vi "Aufschaltung CalGas Span.vi"(4 "Status Str Referenz":refnum<vi>, 6 "Sprachliste":string[][](array[string]), 7 "GD SPAN Eingänge":i32, 8 "error in (no error)":errorcluster caption="Fehler (Eingang, kein Fehler)", 9 "Component Index":i32, 10 "SPAN Index":i32, 11 "SpanInletClusterArray":T1[](array[typedef]) {"zusätzliche Zeitdauer Erster Punkt" min=30 step=1 format="%#_5g"; "Zeitdauer Stufen" format="%#_5g"; "Max Fehler" format="%#_5g"; "Anzahl Stufen" format="%#_5g"; "Komponenten"."Komponente 5"."Komponente:" items=["NO (350,3000) LP 191C", "NO2 (150) LP 191C (1of2)", "NO2 (2000) LP 191C (2of2)", "N2O (300) LP 191C (1of2)", "NH3 (300) LP 191C (1of2)", "NH3 (900,3000) LP 191C (2of2)", "HNCO (400) 191C", "H2O% (30) LP 191C", "Formaldehyde (70,500) LP 191C", "CO2 low% (4) LP 191C (2of2)", "CO2% (20) LP 191C (1of2)", "CO (700) LP 191C (1of3)", "CO% (1) LP 191C (2of3)", "Propylene (1000) LP 191C", "Aromatic HC C7 (500) LP 191C", "Ethylene (1000) LP 191C", "CH4 (250) LP 191C (1of2)", "CH4 (5000) LP 191C (2of2)", "Ethane (1000) LP 191C", "Acetylene (1000) LP 191C", "HNO2 (20) 191C", "MeOH (1000) 191C", "CO% (10) LP 191C (3of3)", "Formic Acid (100) 191C", "SO2 (500) LP 191C", "Acetaldehyde (1000) LP 191C", "COS (100) LP 191C", "1,3 butadiene (100) LP 191C", "Oil as Octane (200) LP 191C", "N2O (1000) LP 191C (2of2)", "Propane (200) LP 191C", "NO2 autorange (2000)", "CO autorange (100000)", "CH4 autorange (5000)", "NH3 autorange (3000)", "Temp. Gascell", "Pressure Gascell", "sBeam@2500"]; "Komponenten"."Komponente 5"."Konzentration IST" format="%#.4f"; "Komponenten"."Komponente 5"."Genauigkeit" format="%#.1f"; "Komponenten"."Komponente 4"."Komponente:" items=["NO (350,3000) LP 191C", "NO2 (150) LP 191C (1of2)", "NO2 (2000) LP 191C (2of2)", "N2O (300) LP 191C (1of2)", "NH3 (300) LP 191C (1of2)", "NH3 (900,3000) LP 191C (2of2)", "HNCO (400) 191C", "H2O% (30) LP 191C", "Formaldehyde (70,500) LP 191C", "CO2 low% (4) LP 191C (2of2)", "CO2% (20) LP 191C (1of2)", "CO (700) LP 191C (1of3)", "CO% (1) LP 191C (2of3)", "Propylene (1000) LP 191C", "Aromatic HC C7 (500) LP 191C", "Ethylene (1000) LP 191C", "CH4 (250) LP 191C (1of2)", "CH4 (5000) LP 191C (2of2)", "Ethane (1000) LP 191C", "Acetylene (1000) LP 191C", "HNO2 (20) 191C", "MeOH (1000) 191C", "CO% (10) LP 191C (3of3)", "Formic Acid (100) 191C", "SO2 (500) LP 191C", "Acetaldehyde (1000) LP 191C", "COS (100) LP 191C", "1,3 butadiene (100) LP 191C", "Oil as Octane (200) LP 191C", "N2O (1000) LP 191C (2of2)", "Propane (200) LP 191C", "NO2 autorange (2000)", "CO autorange (100000)", "CH4 autorange (5000)", "NH3 autorange (3000)", "Temp. Gascell", "Pressure Gascell", "sBeam@2500"]; "Komponenten"."Komponente 4"."Konzentration IST" format="%#.4f"; "Komponenten"."Komponente 4"."Genauigkeit" format="%#.1f"; "Komponenten"."Komponente 3"."Komponente:" items=["NO (350,3000) LP 191C", "NO2 (150) LP 191C (1of2)", "NO2 (2000) LP 191C (2of2)", "N2O (300) LP 191C (1of2)", "NH3 (300) LP 191C (1of2)", "NH3 (900,3000) LP 191C (2of2)", "HNCO (400) 191C", "H2O% (30) LP 191C", "Formaldehyde (70,500) LP 191C", "CO2 low% (4) LP 191C (2of2)", "CO2% (20) LP 191C (1of2)", "CO (700) LP 191C (1of3)", "CO% (1) LP 191C (2of3)", "Propylene (1000) LP 191C", "Aromatic HC C7 (500) LP 191C", "Ethylene (1000) LP 191C", "CH4 (250) LP 191C (1of2)", "CH4 (5000) LP 191C (2of2)", "Ethane (1000) LP 191C", "Acetylene (1000) LP 191C", "HNO2 (20) 191C", "MeOH (1000) 191C", "CO% (10) LP 191C (3of3)", "Formic Acid (100) 191C", "SO2 (500) LP 191C", "Acetaldehyde (1000) LP 191C", "COS (100) LP 191C", "1,3 butadiene (100) LP 191C", "Oil as Octane (200) LP 191C", "N2O (1000) LP 191C (2of2)", "Propane (200) LP 191C", "NO2 autorange (2000)", "CO autorange (100000)", "CH4 autorange (5000)", "NH3 autorange (3000)", "Temp. Gascell", "Pressure Gascell", "sBeam@2500"]; "Komponenten"."Komponente 3"."Konzentration IST" format="%#.4f"; "Komponenten"."Komponente 3"."Genauigkeit" format="%#.1f"; "Komponenten"."Komponente 2"."Komponente:" items=["NO (350,3000) LP 191C", "NO2 (150) LP 191C (1of2)", "NO2 (2000) LP 191C (2of2)", "N2O (300) LP 191C (1of2)", "NH3 (300) LP 191C (1of2)", "NH3 (900,3000) LP 191C (2of2)", "HNCO (400) 191C", "H2O% (30) LP 191C", "Formaldehyde (70,500) LP 191C", "CO2 low% (4) LP 191C (2of2)", "CO2% (20) LP 191C (1of2)", "CO (700) LP 191C (1of3)", "CO% (1) LP 191C (2of3)", "Propylene (1000) LP 191C", "Aromatic HC C7 (500) LP 191C", "Ethylene (1000) LP 191C", "CH4 (250) LP 191C (1of2)", "CH4 (5000) LP 191C (2of2)", "Ethane (1000) LP 191C", "Acetylene (1000) LP 191C", "HNO2 (20) 191C", "MeOH (1000) 191C", "CO% (10) LP 191C (3of3)", "Formic Acid (100) 191C", "SO2 (500) LP 191C", "Acetaldehyde (1000) LP 191C", "COS (100) LP 191C", "1,3 butadiene (100) LP 191C", "Oil as Octane (200) LP 191C", "N2O (1000) LP 191C (2of2)", "Propane (200) LP 191C", "NO2 autorange (2000)", "CO autorange (100000)", "CH4 autorange (5000)", "NH3 autorange (3000)", "Temp. Gascell", "Pressure Gascell", "sBeam@2500"]; "Komponenten"."Komponente 2"."Konzentration IST" format="%#.4f"; "Komponenten"."Komponente 2"."Genauigkeit" format="%#.1f"; "Komponenten"."Komponente 1"."Komponente:" items=["NO (350,3000) LP 191C", "NO2 (150) LP 191C (1of2)", "NO2 (2000) LP 191C (2of2)", "N2O (300) LP 191C (1of2)", "NH3 (300) LP 191C (1of2)", "NH3 (900,3000) LP 191C (2of2)", "HNCO (400) 191C", "H2O% (30) LP 191C", "Formaldehyde (70,500) LP 191C", "CO2 low% (4) LP 191C (2of2)", "CO2% (20) LP 191C (1of2)", "CO (700) LP 191C (1of3)", "CO% (1) LP 191C (2of3)", "Propylene (1000) LP 191C", "Aromatic HC C7 (500) LP 191C", "Ethylene (1000) LP 191C", "CH4 (250) LP 191C (1of2)", "CH4 (5000) LP 191C (2of2)", "Ethane (1000) LP 191C", "Acetylene (1000) LP 191C", "HNO2 (20) 191C", "MeOH (1000) 191C", "CO% (10) LP 191C (3of3)", "Formic Acid (100) 191C", "SO2 (500) LP 191C", "Acetaldehyde (1000) LP 191C", "COS (100) LP 191C", "1,3 butadiene (100) LP 191C", "Oil as Octane (200) LP 191C", "N2O (1000) LP 191C (2of2)", "Propane (200) LP 191C", "NO2 autorange (2000)", "CO autorange (100000)", "CH4 autorange (5000)", "NH3 autorange (3000)", "Temp. Gascell", "Pressure Gascell", "sBeam@2500"]; "Komponenten"."Komponente 1"."Konzentration IST" format="%#.4f"; "Komponenten"."Komponente 1"."Genauigkeit" format="%#.1f"; "Ablaufdatum" format="%<%d.%m.%Y>T"; "Gasflasche" items=["----"=10000, "IAG NH3 3000"=0, "IAG NH3 200"=1, "IAG NH3 2000"=2, "IAG MG"=3, "IAG O2"=4]}) -> (0 "error out":errorcluster caption="Fehler (Ausgang)", 1 "Status out":string, 2 "SPAN Index out":i32, 3 "SpanInletClusterArray out":T1[](array[typedef]) {"zusätzliche Zeitdauer Erster Punkt" min=30 step=1 format="%#_5g"; "Zeitdauer Stufen" format="%#_5g"; "Max Fehler" format="%#_5g"; "Anzahl Stufen" format="%#_5g"; "Komponenten"."Komponente 5"."Komponente:" items=["NO (350,3000) LP 191C", "NO2 (150) LP 191C (1of2)", "NO2 (2000) LP 191C (2of2)", "N2O (300) LP 191C (1of2)", "NH3 (300) LP 191C (1of2)", "NH3 (900,3000) LP 191C (2of2)", "HNCO (400) 191C", "H2O% (30) LP 191C", "Formaldehyde (70,500) LP 191C", "CO2 low% (4) LP 191C (2of2)", "CO2% (20) LP 191C (1of2)", "CO (700) LP 191C (1of3)", "CO% (1) LP 191C (2of3)", "Propylene (1000) LP 191C", "Aromatic HC C7 (500) LP 191C", "Ethylene (1000) LP 191C", "CH4 (250) LP 191C (1of2)", "CH4 (5000) LP 191C (2of2)", "Ethane (1000) LP 191C", "Acetylene (1000) LP 191C", "HNO2 (20) 191C", "MeOH (1000) 191C", "CO% (10) LP 191C (3of3)", "Formic Acid (100) 191C", "SO2 (500) LP 191C", "Acetaldehyde (1000) LP 191C", "COS (100) LP 191C", "1,3 butadiene (100) LP 191C", "Oil as Octane (200) LP 191C", "N2O (1000) LP 191C (2of2)", "Propane (200) LP 191C", "NO2 autorange (2000)", "CO autorange (100000)", "CH4 autorange (5000)", "NH3 autorange (3000)", "Temp. Gascell", "Pressure Gascell", "sBeam@2500"]; "Komponenten"."Komponente 5"."Konzentration IST" format="%#.4f"; "Komponenten"."Komponente 5"."Genauigkeit" format="%#.1f"; "Komponenten"."Komponente 4"."Komponente:" items=["NO (350,3000) LP 191C", "NO2 (150) LP 191C (1of2)", "NO2 (2000) LP 191C (2of2)", "N2O (300) LP 191C (1of2)", "NH3 (300) LP 191C (1of2)", "NH3 (900,3000) LP 191C (2of2)", "HNCO (400) 191C", "H2O% (30) LP 191C", "Formaldehyde (70,500) LP 191C", "CO2 low% (4) LP 191C (2of2)", "CO2% (20) LP 191C (1of2)", "CO (700) LP 191C (1of3)", "CO% (1) LP 191C (2of3)", "Propylene (1000) LP 191C", "Aromatic HC C7 (500) LP 191C", "Ethylene (1000) LP 191C", "CH4 (250) LP 191C (1of2)", "CH4 (5000) LP 191C (2of2)", "Ethane (1000) LP 191C", "Acetylene (1000) LP 191C", "HNO2 (20) 191C", "MeOH (1000) 191C", "CO% (10) LP 191C (3of3)", "Formic Acid (100) 191C", "SO2 (500) LP 191C", "Acetaldehyde (1000) LP 191C", "COS (100) LP 191C", "1,3 butadiene (100) LP 191C", "Oil as Octane (200) LP 191C", "N2O (1000) LP 191C (2of2)", "Propane (200) LP 191C", "NO2 autorange (2000)", "CO autorange (100000)", "CH4 autorange (5000)", "NH3 autorange (3000)", "Temp. Gascell", "Pressure Gascell", "sBeam@2500"]; "Komponenten"."Komponente 4"."Konzentration IST" format="%#.4f"; "Komponenten"."Komponente 4"."Genauigkeit" format="%#.1f"; "Komponenten"."Komponente 3"."Komponente:" items=["NO (350,3000) LP 191C", "NO2 (150) LP 191C (1of2)", "NO2 (2000) LP 191C (2of2)", "N2O (300) LP 191C (1of2)", "NH3 (300) LP 191C (1of2)", "NH3 (900,3000) LP 191C (2of2)", "HNCO (400) 191C", "H2O% (30) LP 191C", "Formaldehyde (70,500) LP 191C", "CO2 low% (4) LP 191C (2of2)", "CO2% (20) LP 191C (1of2)", "CO (700) LP 191C (1of3)", "CO% (1) LP 191C (2of3)", "Propylene (1000) LP 191C", "Aromatic HC C7 (500) LP 191C", "Ethylene (1000) LP 191C", "CH4 (250) LP 191C (1of2)", "CH4 (5000) LP 191C (2of2)", "Ethane (1000) LP 191C", "Acetylene (1000) LP 191C", "HNO2 (20) 191C", "MeOH (1000) 191C", "CO% (10) LP 191C (3of3)", "Formic Acid (100) 191C", "SO2 (500) LP 191C", "Acetaldehyde (1000) LP 191C", "COS (100) LP 191C", "1,3 butadiene (100) LP 191C", "Oil as Octane (200) LP 191C", "N2O (1000) LP 191C (2of2)", "Propane (200) LP 191C", "NO2 autorange (2000)", "CO autorange (100000)", "CH4 autorange (5000)", "NH3 autorange (3000)", "Temp. Gascell", "Pressure Gascell", "sBeam@2500"]; "Komponenten"."Komponente 3"."Konzentration IST" format="%#.4f"; "Komponenten"."Komponente 3"."Genauigkeit" format="%#.1f"; "Komponenten"."Komponente 2"."Komponente:" items=["NO (350,3000) LP 191C", "NO2 (150) LP 191C (1of2)", "NO2 (2000) LP 191C (2of2)", "N2O (300) LP 191C (1of2)", "NH3 (300) LP 191C (1of2)", "NH3 (900,3000) LP 191C (2of2)", "HNCO (400) 191C", "H2O% (30) LP 191C", "Formaldehyde (70,500) LP 191C", "CO2 low% (4) LP 191C (2of2)", "CO2% (20) LP 191C (1of2)", "CO (700) LP 191C (1of3)", "CO% (1) LP 191C (2of3)", "Propylene (1000) LP 191C", "Aromatic HC C7 (500) LP 191C", "Ethylene (1000) LP 191C", "CH4 (250) LP 191C (1of2)", "CH4 (5000) LP 191C (2of2)", "Ethane (1000) LP 191C", "Acetylene (1000) LP 191C", "HNO2 (20) 191C", "MeOH (1000) 191C", "CO% (10) LP 191C (3of3)", "Formic Acid (100) 191C", "SO2 (500) LP 191C", "Acetaldehyde (1000) LP 191C", "COS (100) LP 191C", "1,3 butadiene (100) LP 191C", "Oil as Octane (200) LP 191C", "N2O (1000) LP 191C (2of2)", "Propane (200) LP 191C", "NO2 autorange (2000)", "CO autorange (100000)", "CH4 autorange (5000)", "NH3 autorange (3000)", "Temp. Gascell", "Pressure Gascell", "sBeam@2500"]; "Komponenten"."Komponente 2"."Konzentration IST" format="%#.4f"; "Komponenten"."Komponente 2"."Genauigkeit" format="%#.1f"; "Komponenten"."Komponente 1"."Komponente:" items=["NO (350,3000) LP 191C", "NO2 (150) LP 191C (1of2)", "NO2 (2000) LP 191C (2of2)", "N2O (300) LP 191C (1of2)", "NH3 (300) LP 191C (1of2)", "NH3 (900,3000) LP 191C (2of2)", "HNCO (400) 191C", "H2O% (30) LP 191C", "Formaldehyde (70,500) LP 191C", "CO2 low% (4) LP 191C (2of2)", "CO2% (20) LP 191C (1of2)", "CO (700) LP 191C (1of3)", "CO% (1) LP 191C (2of3)", "Propylene (1000) LP 191C", "Aromatic HC C7 (500) LP 191C", "Ethylene (1000) LP 191C", "CH4 (250) LP 191C (1of2)", "CH4 (5000) LP 191C (2of2)", "Ethane (1000) LP 191C", "Acetylene (1000) LP 191C", "HNO2 (20) 191C", "MeOH (1000) 191C", "CO% (10) LP 191C (3of3)", "Formic Acid (100) 191C", "SO2 (500) LP 191C", "Acetaldehyde (1000) LP 191C", "COS (100) LP 191C", "1,3 butadiene (100) LP 191C", "Oil as Octane (200) LP 191C", "N2O (1000) LP 191C (2of2)", "Propane (200) LP 191C", "NO2 autorange (2000)", "CO autorange (100000)", "CH4 autorange (5000)", "NH3 autorange (3000)", "Temp. Gascell", "Pressure Gascell", "sBeam@2500"]; "Komponenten"."Komponente 1"."Konzentration IST" format="%#.4f"; "Komponenten"."Komponente 1"."Genauigkeit" format="%#.1f"; "Ablaufdatum" format="%<%d.%m.%Y>T"; "Gasflasche" items=["----"=10000, "IAG NH3 3000"=0, "IAG NH3 200"=1, "IAG NH3 2000"=2, "IAG MG"=3, "IAG O2"=4]})   [LabVIEW 2020, in "Linearisierung v2.lvlib" / "SpanEinstellungen.lvlib"]
uses:
  SpanEinstellungen.lvlib
  SpanInletCluster.ctl
  Seiten/System Einstellungen V2/Konfig Gasflasche.ctl
  Seiten/System Einstellungen V2/Analysatoren.ctl
  Seiten/System Einstellungen V2/Gasflasche Auswahl.ctl
  Komponentencluster mit Formel.ctl
  Komponentenauswahl mit Formel.ctl
  Visualisierungs Elemente/String - Eingabefeld.ctl
  Einheit.ctl
  Seiten/System Einstellungen V2/Traegergas.ctl
  Aktion Lin Daten aufarbeiten.ctl
  Visualisierungs Elemente/Zahlen-Eingabefeld.ctl
  Seiten/CalGas Aufschaltung/FGV CalGas Aktionen.ctl
  Seiten/CalGas Aufschaltung/Auswahl Aufschaltpunkt.ctl
  Gasteiler/Aktionen FGV Gasteiler Daten.ctl
  Aktion FGV GD Errors sammeln.ctl
  GD Info Cluster.ctl
  LIN ErrorCluster.ctl
  Gasteiler/AK-Komm Gasteiler/Aktionen AK Komm.ctl
  Gasteiler/HovaCAL_Interface/Kommunikation/Aktion_FGV_HovaCAL_Interface_GetData.ctl
  Gasteiler/HovaCAL_Interface/Kommunikation/Aktion FGV HovaCAL Interface Autolin.ctl
  Kalibrier Info Cluster.ctl
  Funktionstasten/Funktionstasten-Aktion.ctl
  Funktionstasten/Zustaende.ctl
  Seiten/EL3000/FID/FID Kalibrierung/FID Kalibrieren.ctl
  Seiten/EL3000/PMA/Kalibrieren/Kalibrierung O2.ctl
  Seiten/CalGas Aufschaltung/CalGas Aufschaltung.lvlib
  Seiten/System Einstellungen V2/System Einstellungen V2.lvlib
  Gasteiler/AK-Komm Gasteiler/Alter Gasteiler/Alter Gasteiler.lvlib
  Gasteiler/AK-Komm Gasteiler/Alter Gasteiler/Aktionen AK Komm_ALT.ctl
  Gasteiler/AK-Komm Gasteiler/AK Komm Gasteiler.lvlib
  Gasteiler/Horiba/Aktion Befehl.ctl
  Gasteiler/Horiba/Horiba GDC.lvlib
  Gasteiler/Gasteiler.lvlib
  Linearisierung v2.lvlib
  Funktionstasten/Funktionstasten.lvlib
  Seiten/EL3000/PMA/Kalibrieren/Kalibrieren.lvlib
  Seiten/EL3000/Allgemeine VI/Allgemeine VI.lvlib
  Seiten/EL3000/FID/FID Kalibrierung/FID Kalibrierung.lvlib
  Gasteiler/HovaCAL_Interface/Kommunikation/Kommunikation.lvlib
panel:
  # "sec"
  # "%"
  # "sec"
  # "Komponente"
  # "Formel"
  # "Konzentration"
  # "Einheit"
  # "Genauigkeit [%]"
  # "sec"
  # "%"
  # "sec"
  # "Komponente"
  # "Formel"
  # "Konzentration"
  # "Einheit"
  # "Genauigkeit [%]"
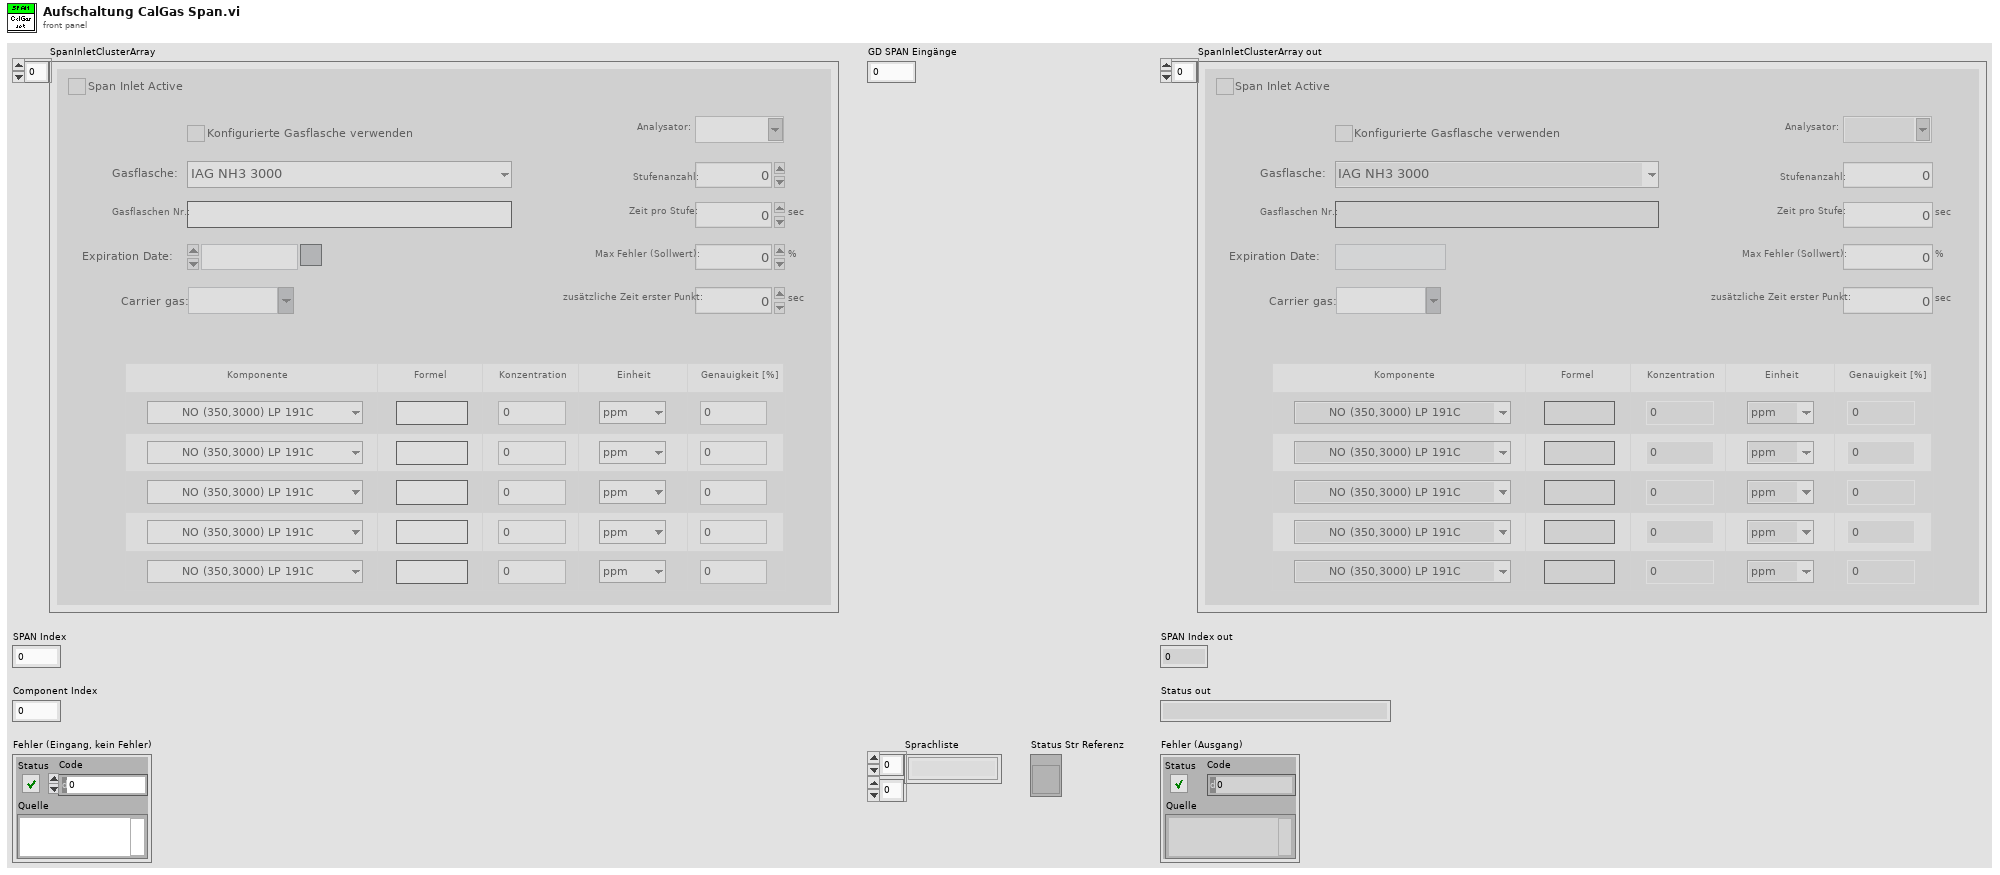
[diagram p1: front panel]
types:
  T1 = typedef "Linearisierung v2.lvlib/SpanEinstellungen.lvlib/SpanInletCluster.ctl" = cluster{"Span Inlet Active":T2, "Analysator":T3, "Konfig Gasflasche":T2, "Gasflasche":T4, "Gasflaschen Nr.:":string, "Ablaufdatum":timestamp, "Komponenten":T5, "Zeitdauer Stufen":sgl, "Max Fehler":sgl, "Anzahl Stufen":sgl, "Trägergas":T9, "zusätzliche Zeitdauer Erster Punkt":sgl}
  T2 = typedef "System Einstellungen V2.lvlib/Konfig Gasflasche.ctl" = bool
  T3 = typedef "System Einstellungen V2.lvlib/Analysatoren.ctl" = string
  T4 = typedef "System Einstellungen V2.lvlib/Gasflasche Auswahl.ctl" = u16
  T5 = typedef "Linearisierung v2.lvlib/SpanEinstellungen.lvlib/Komponentencluster mit Formel.ctl" = cluster{"Komponente 1":T6, "Komponente 2":T6, "Komponente 3":T6, "Komponente 4":T6, "Komponente 5":T6}
  T6 = typedef "Linearisierung v2.lvlib/SpanEinstellungen.lvlib/Komponentenauswahl mit Formel.ctl" = cluster{"Komponente:":u16, "Summenformel":T7, "Konzentration IST":dbl, "Einheit":T8, "Genauigkeit":dbl}
  T7 = typedef "String - Eingabefeld.ctl" = string
  T8 = typedef "Linearisierung v2.lvlib/SpanEinstellungen.lvlib/Einheit.ctl" = enum16{"ppm", "%"}
  T9 = typedef "System Einstellungen V2.lvlib/Traegergas.ctl" = string
  T10 = typedef "Zahlen-Eingabefeld.ctl" = sgl
  T11 = typedef "Linearisierung v2.lvlib/Aktion Lin Daten aufarbeiten.ctl" = enum16{"lesen", "Protkolldaten", "speichern", "laden", "EPA auswerten", "Tabelle schreiben", "Lin auswerten", "Tab init", "Stufentabelle", "EPA aktiviert", "Nachbehandlung laden", "Tabelle löschen", "Istwerte löschen", "Zeile löschen", "Zeile einfügen", "LIN aktiviert", "LIN/EPA aktiv laden", "EGAK Tab", "LIN übernehmen", "Tab init ohne Stufen"}
  T12 = typedef "Linearisierung v2.lvlib/Lin-Polynom Daten.ctl" = cluster{"Messgerät":string, "Kalibrator (Gasteiler)":string, "Bearbeiter/in":string, "Komponente":string, "Zeitstempel":timestamp, "F_max gefordert (%)":sgl, "F_max in %":sgl, "F_max in ppm":sgl, "Vorschlag Ordnung":i32, "Polynom OK":bool, "Polynomkoeff.":dbl[], "Prüfgas Konzentration":dbl, "Pfad EPA":string, "Pfad_LIN":string, "Gasnummer:":u8, "Komponentenauswahl":T13, "Verdünnungsgas":T15, "Zeitdauer Stufe":T10, "Anzahl Stufen":T10, "F_max in % EPA":sgl, "F_max in ppm EPA":sgl, "F_max in % LIN":sgl, "F_max in ppm LIN":sgl, "Punkte umkehren":bool, "EPA Optionsfeld":T16, "Autolin Hovacal":T17, "Spanfactors":sgl[], "Kalibrierauswahl":T18, "Conditions:":T19, "Gasflaschen Nr.:":string, "Bottle Accuracy":dbl, "Konfig Gasflasche":T2, "Gasflasche":T4, "HovaCAL Flow AutoLin":T20, "MFC Output":T21, "Gas Ablaufdatum":timestamp, "Lin Modus":T22, "zusätzliche Zeitdauer Erster Punkt":sgl, "Offsets":sgl[]}
  T13 = typedef "Linearisierung v2.lvlib/KomponentenArray.ctl" = cluster{"Komponente:":T14, "Konzentration":dbl}[]
  T14 = typedef "Auswahlfeld.ctl" = u16
  T15 = typedef "Linearisierung v2.lvlib/Gasteiler.lvlib/Prüfgas in.ctl" = u16
  T16 = typedef "Linearisierung v2.lvlib/EPA Optionsfeld.ctl" = enum32{"Istwert", "Rohwert", "Linearisierter Wert"}
  T17 = typedef "Linearisierung v2.lvlib/Gasteiler.lvlib/HovaCal.lvlib/AutoLin Hovacal.ctl" = enum32{"Keine Auswahl", "Optionsauswahl 1", "Optionsauswahl 2"}
  T18 = typedef "Linearisierung v2.lvlib/Kalibrieroption.ctl" = u16
  T19 = typedef "Linearisierung v2.lvlib/Linearity verification 1065-307.lvlib/Condition.ctl" = u16
  T20 = typedef "Linearisierung v2.lvlib/Gasteiler.lvlib/HovaCAL_Interface.lvlib/Controls.lvlib/Flow Einstellung.ctl" = cluster{"HovaCAL Flow Input Cluster":dbl}
  T21 = typedef "Linearisierung v2.lvlib/Gasteiler.lvlib/HovaCAL_Interface.lvlib/Controls.lvlib/Pump state.ctl" = cluster{"Run":bool}
  T22 = typedef "CalGas Aufschaltung.lvlib/Lin Modus.ctl" = u16
  T23 = typedef "CalGas Aufschaltung.lvlib/FGV CalGas Aktionen.ctl" = enum16{"lesen", "Analysator Auswahl", "Def.CalGas", "Aufschaltung CalGas", "laden", "speichern", "KAL extrahieren"}
  T24 = typedef "CalGas Aufschaltung.lvlib/Auswahl Aufschaltpunkt.ctl" = enum16{"über Filterblock", "Analysator direkt", "über PNS", "Entnahme", "Gasdivider"}
  T25 = typedef "Linearisierung v2.lvlib/SpanEinstellungen.lvlib/GD Info Cluster.ctl" = cluster{"Wobei":string, "Status":string, "Errors":T26, "Empfangsdaten":string[], "Zeitstempel":string}
  T26 = typedef "Linearisierung v2.lvlib/LIN ErrorCluster.ctl" = cluster{"Störung Kommunikation":bool, "Pressure carrier gas":bool, "Pressure diluted gas":bool, "Outlet Pressure":bool, "SNOX before SAIR":bool, "Störung Gasteiler":bool}
  T27 = typedef "Linearisierung v2.lvlib/SpanEinstellungen.lvlib/Aktion FGV GD Errors sammeln.ctl" = enum16{"lesen", "init", "GD Infos sammeln", "Kalibrierinfos sammeln", "Test Data", "GD Infos selektiv sammeln"}
  T28 = typedef "Linearisierung v2.lvlib/Gasteiler.lvlib/Aktionen FGV Gasteiler Daten.ctl" = enum16{"lesen", "Gasteiler Daten", "Seriellen Param.", "MB-Endwert", "laden", "speichern", "Anforderung", "TCP", "Aufzeichnung Start"}
  T29 = typedef "Linearisierung v2.lvlib/Gasteiler.lvlib/AK Komm Gasteiler.lvlib/Aktionen AK Komm.ctl" = enum16{"lesen", "initialisieren", "beenden", "Status", "SMAN", "SREM", "STBY", "ASTF", "ASTZ", "SLST", "AGAT", "EGAK", "AGAK", "AKAK", "ADRU", "SKOP", "SVSA", "SVSZ", "SONO", "SAIR", "SNOX", "ANOX", "SSPL", "SRUC", "SLIN", "ALST", "ETYP", "SVIO", "LCYL", "CCYL", "DCYL", "SCYL", "GCYL", "DRGV", "DRDC"}
  T30 = typedef "Linearisierung v2.lvlib/Gasteiler.lvlib/AK Komm Gasteiler.lvlib/Alter Gasteiler.lvlib/Aktionen AK Komm_ALT.ctl" = enum16{"lesen", "initialisieren", "beenden", "SRES", "STBY", "SREM", "SMAN", "SLIN", "SLCH", "SLST", "SSPL", "AGAT", "ALST", "ASTZ", "ASTF", "AGAK", "EGAK"}
  T31 = typedef "Linearisierung v2.lvlib/Gasteiler.lvlib/Horiba GDC.lvlib/Aktion Befehl.ctl" = enum16{"lesen", "initialisieren", "Beenden", "Standby", "GD/CC", "Info", "Flow", "Alarm", "GD parameter", "GD point", "Durchfluss", "Spuelen1", "Spuelen1 On", "Spuelen1Off", "Spuelen2", "Ventil-Abfrage", "Reset"}
  T32 = typedef "Linearisierung v2.lvlib/Gasteiler.lvlib/HovaCAL_Interface.lvlib/Kommunikation.lvlib/Aktion_FGV_HovaCAL_Interface_GetData.ctl" = enum16{"lesen", "SystemInfo", "MFC Info", "actual Values", "Limits", "first contact"}
  T33 = typedef "Linearisierung v2.lvlib/Gasteiler.lvlib/HovaCAL_Interface.lvlib/Kommunikation.lvlib/Aktion FGV HovaCAL Interface Autolin.ctl" = enum16{"lesen", "schreiben", "MFC Komponente fix setzen", "init"}
  T34 = typedef "CalGas Aufschaltung.lvlib/Aufschaltung CalGas.ctl" = cluster{"Kalibriergas":T14, "Aufschaltpunkt":T24, "Analysator":T35}
  T35 = typedef "CalGas Aufschaltung.lvlib/Auswahl Analysator.ctl" = enum16{"FT-IR", "FID", "PMA", "PMA/FID/FT-IR"}
  T36 = typedef "Linearisierung v2.lvlib/GasteilerType.ctl" = u16
  T37 = typedef "Linearisierung v2.lvlib/Gasteiler.lvlib/Gasteiler Fehler.ctl" = cluster{"Pressure carrier gas":bool, "Pressure diluted gas":bool, "Outlet Pressure":bool, "SNOX before SAIR":bool}
  T38 = typedef "Linearisierung v2.lvlib/Gasteiler.lvlib/HovaCAL_Interface.lvlib/Controls.lvlib/Info Cluster.ctl" = cluster{"device":string, "version":string, "number of mfc":i32, "number of pumps":i32, "number of temp controllers":i32, "number of mfs":i32, "number of balances":i32}
  T39 = typedef "Funktionstasten.lvlib/Zustaende.ctl" = enum16{"Standby", "Pause", "Eco", "Messen", "Kalibrieren", "Spülen Filter", "Spülen Leitung", "Umgebungsluft", "0-Gas", "Cal-Gas", "CG zu PNS", "-------------", "Init 1", "Init 2", "Init 3", "Init 4", "Messen vorbereiten", "Messen durchführen", "Exit"}
  T40 = typedef "Funktionstasten.lvlib/Funktionstasten-Aktion.ctl" = enum16{"Initialisieren", "Zustand setzen", "Taste gedrückt", "Fehler speichern", "Lesen", "Manuell", "Remote", "Bitparallel", "Samplepoint", "Zeit Prüfen", "reset Umschalten"}
  T41 = typedef "ABB-EL3000.lvlib/FID.lvlib/FID Kalibrierung.lvlib/FID Kalibrieren.ctl" = enum16{"CH4 Nullpunkt", "THC Nullpunkt", "NMHC Nullpunkt", "CH4 Endpunkt", "THC Endpunkt", "NMHC Endpunkt"}
  T42 = typedef "ABB-EL3000.lvlib/PMA.lvlib/Kalibrieren.lvlib/Kalibrierung O2.ctl" = enum16{"Nullpunkt O2", "Endpunkt O2"}
  T43 = typedef "Linearisierung v2.lvlib/SpanEinstellungen.lvlib/Kalibrier Info Cluster.ctl" = cluster{"Wobei":string, "Calibration succesful":bool, "Value is in the valid range":bool, "Zeitstempel":string}
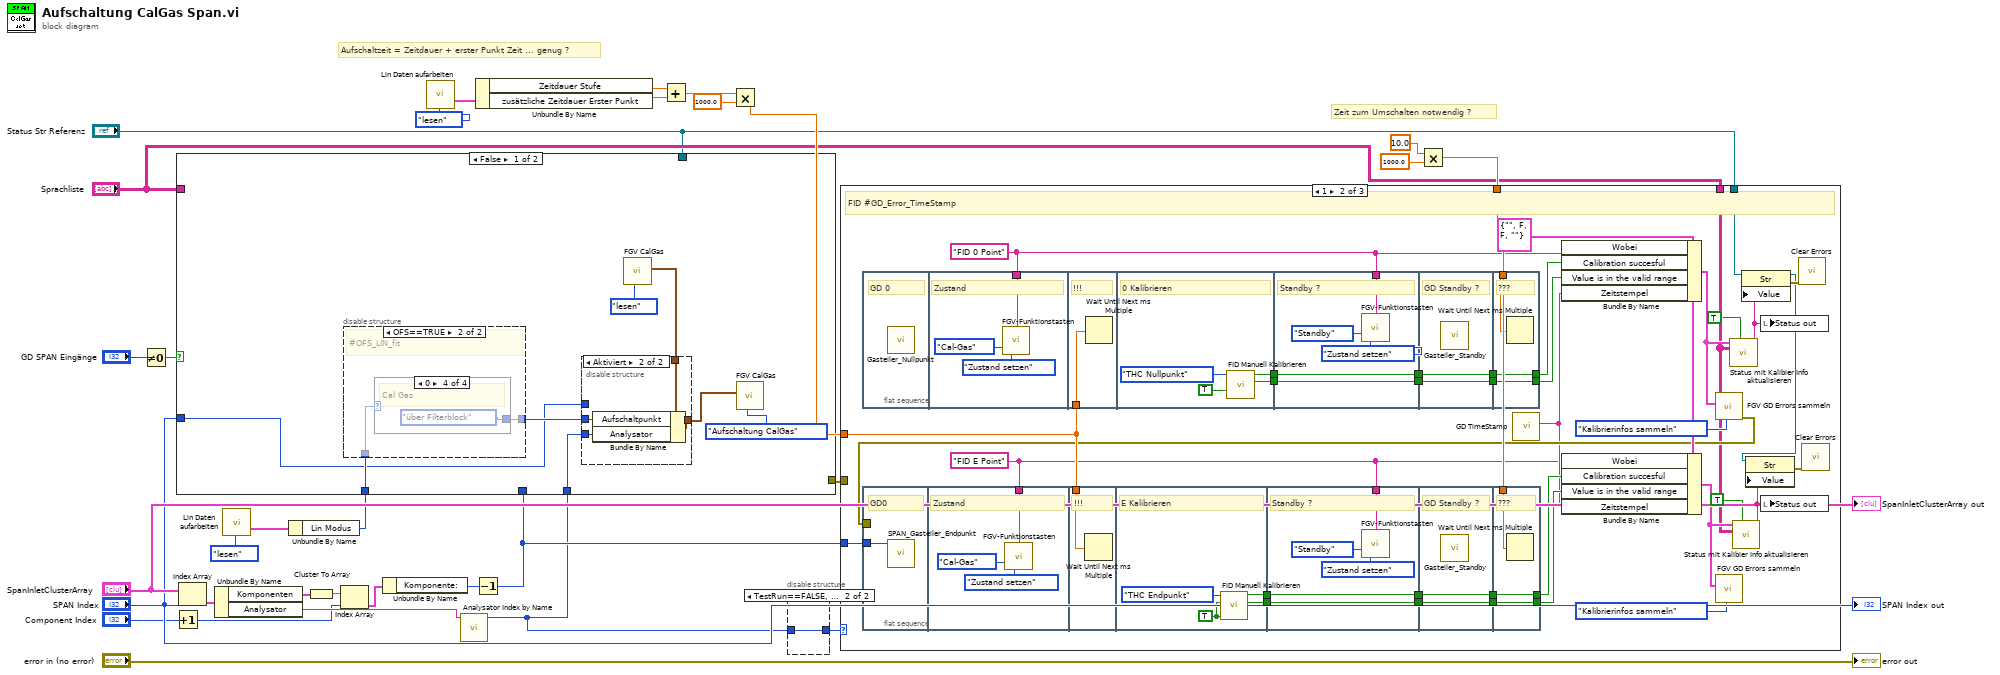
[diagram p0: block diagram]
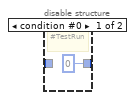
[diagram p2: hidden frame]
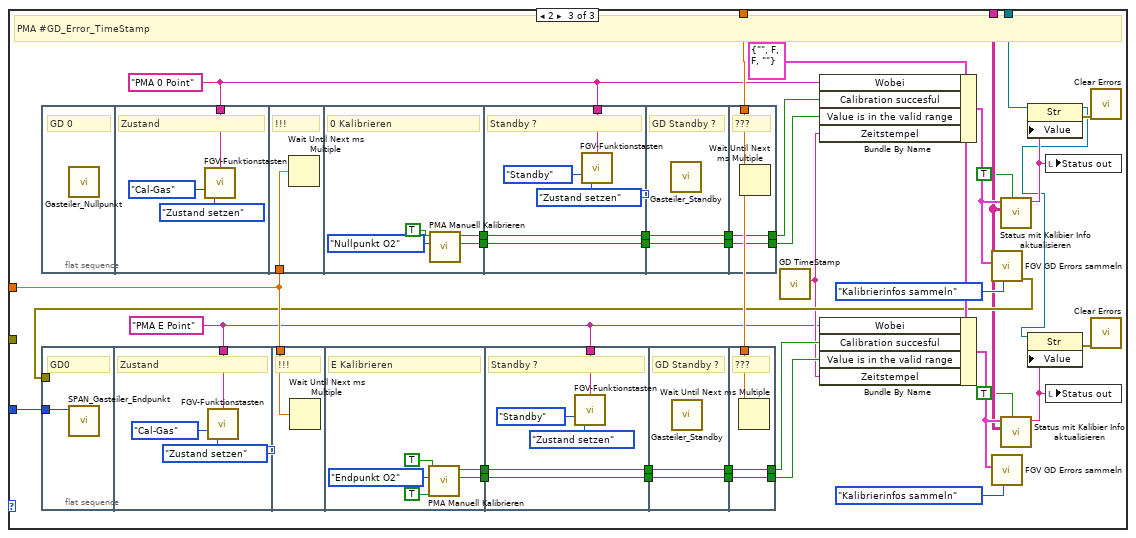
[diagram p4: hidden frame]
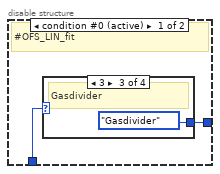
[diagram p5: hidden frame]
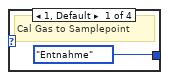
[diagram p6: hidden frame]
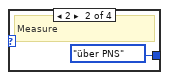
[diagram p7: hidden frame]
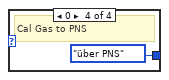
[diagram p8: hidden frame]
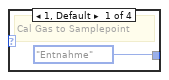
[diagram p9: hidden frame]
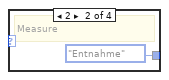
[diagram p10: hidden frame]
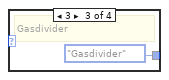
[diagram p11: hidden frame]
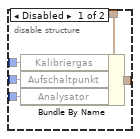
[diagram p12: hidden frame]
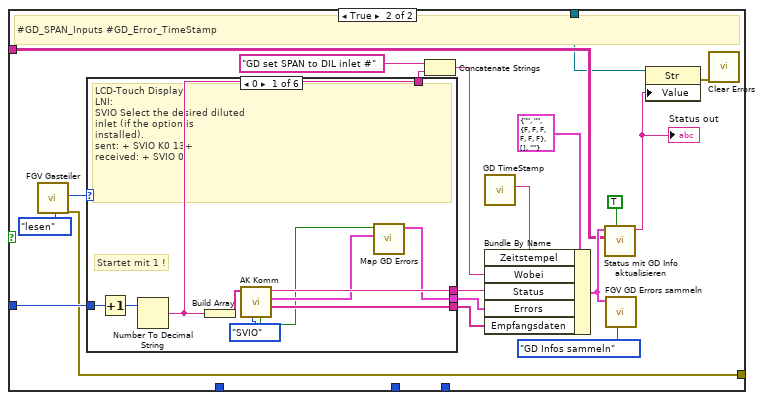
[diagram p13: hidden frame]
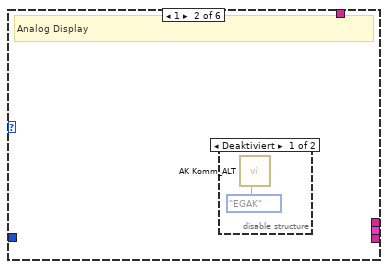
[diagram p14: hidden frame]
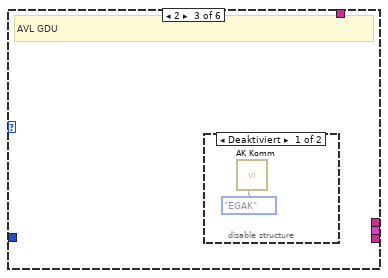
[diagram p16: hidden frame]
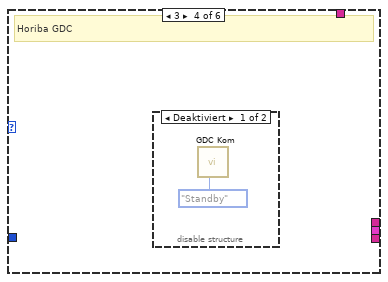
[diagram p18: hidden frame]
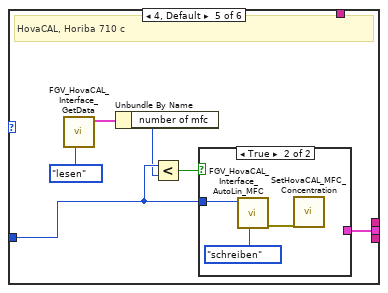
[diagram p20: hidden frame]
diagram:
  # "Zeit zum Umschalten notwendig ?"
  # "Aufschaltzeit = Zeitdauer + erster Punkt Zeit ... genug ?"
  n1 = Not Equal To 0?(x="GD SPAN Eingänge") -> (x != 0?=w28:bool)
  n2 = Increment(x="Component Index") -> (x+1=w17:i32)
  n3 = Index Array(array="SpanInletClusterArray", index="SPAN Index") -> (element=w23:T1)
  n4 = Unbundle By Name(w23) -> ("Komponenten"=w21:T5, "Analysator"=w31:T3)
  n5 = call "Lin Daten aufarbeiten.vi"("Aktionen"=Aktion_Lin_Daten_aufarbeiten."lesen") -> ("Lin-Polynom"=w26:T12)  [unwired: 16 in, 10 out]
  n6 = Unbundle By Name(w26) -> ("Lin Modus"=w2:T22)
  n7 = Cluster To Array(cluster=w21) -> (array=w22:T6[])
  n8 = Index Array(array=w22, index=w17) -> (element=w19:T6)
  n9 = Unbundle By Name(w19) -> ("Komponente:"=w18:u16)
  n10 = call "Lin Daten aufarbeiten.vi"("Aktionen"=Aktion_Lin_Daten_aufarbeiten."lesen") -> ("Lin-Polynom"=w14:T12)  [unwired: 16 in, 10 out]
  n11 = call "Analysator Index by Name.vi"("Analysator"=w31) -> ("Analysator Index"=w1:i32)  [unwired: 10 in]
  n12 = Decrement(x=w18) -> (x-1=w3:u16)
  n13 = case shown="False" w28 {
    tunnel: "SPAN Index" -> [w33 w78]
    tunnel: [_ w77] -> w25
    tunnel: "Sprachliste" -> [_ w69]
    tunnel: "Status Str Referenz" -> [_ w66]
    tunnel: w3 -> [_ _]
    tunnel: w2 -> [w35 _]
    tunnel: w1 -> [w38 _]
    frame False {
      n14 = disable-structure shown="OFS==TRUE" {
        disable-tunnel: w35 -> [w42 w48]
        disable-tunnel: [w41 w47] -> w34
        frame condition #0 (active) {
          # "#OFS_LIN_fit"
          n15 = case shown="3" w42 {
            tunnel: [Auswahl_Aufschaltpunkt."Entnahme" ("Aufschaltpunkt") Auswahl_Aufschaltpunkt."über PNS" ("Aufschaltpunkt") Auswahl_Aufschaltpunkt."Gasdivider" ("Aufschaltpunkt") Auswahl_Aufschaltpunkt."über PNS" ("Aufschaltpunkt")] -> w41
            frame 1, Default {
              # "Cal Gas to Samplepoint"
            }
            frame 2 {
              # "Measure"
            }
            frame 3 {
              # "Gasdivider"
            }
            frame 0 {
              # "Cal Gas to PNS"
            }
          }
        }
        frame condition #1 {
          # "#OFS_LIN_fit"
          n16 = case shown="0" w48 {
            tunnel: [Auswahl_Aufschaltpunkt."Entnahme" ("Aufschaltpunkt") Auswahl_Aufschaltpunkt."Entnahme" ("Aufschaltpunkt") Auswahl_Aufschaltpunkt."Gasdivider" ("Aufschaltpunkt") Auswahl_Aufschaltpunkt."über Filterblock" ("Aufschaltpunkt")] -> w47
            frame 1, Default {
              # "Cal Gas to Samplepoint"
            }
            frame 2 {
              # "Measure"
            }
            frame 3 {
              # "Gasdivider"
            }
            frame 0 {
              # "Cal Gas"
            }
          }
        }
      }
      n17 = call "FGV CalGas.vi"("Aktionen"=FGV_CalGas_Aktionen."lesen") -> ("Aufschaltung CalGas"=w39:T34)  [unwired: 6 in, 4 out]
      n18 = disable-structure shown="Aktiviert" {
        disable-tunnel: [w57 w61] -> w40
        disable-tunnel: w39 -> [w56 w60]
        disable-tunnel: w38 -> [w55 w59]
        disable-tunnel: w34 -> [w54 w58]
        disable-tunnel: w33 -> [w53 _]
        frame Disabled {
          n19 = Bundle By Name(cluster=w56, "Kalibriergas"=w53, "Aufschaltpunkt"=w54, "Analysator"=w55) -> (w57:T34)
        }
        frame Enabled {
          n20 = Bundle By Name(cluster=w60, "Aufschaltpunkt"=w58, "Analysator"=w59) -> (w61:T34)
        }
      }
      n21 = call "FGV CalGas.vi"("Aktionen"=FGV_CalGas_Aktionen."Aufschaltung CalGas", "Aufschaltung CalGas"=w40) -> ()  [unwired: 5 in, 5 out]
    }
    frame True {
      # "#GD_SPAN_Inputs #GD_Error_TimeStamp"
      n22 = call "FGV Gasteiler.vi"("Aktionen"=Aktionen_FGV_Gasteiler_Daten."lesen") -> ("Gasteiler Type"=w79:T36, "error out"=w77:errorcluster)  [unwired: 11 in, 6 out]
      n23 = case shown="0" w79 {
        tunnel: w78 -> [w89 _ _ _ w98 _]
        tunnel: [w86 _ _ _ _ _] -> w74
        tunnel: [w82 _ _ _ w94 _] -> w75
        tunnel: [w85 _ _ _ _ _] -> w76
        tunnel: [w81 _ _ _ _ _] -> w63
        frame 0 {
          # "Startet mit 1 !"
          # "LCD-Touch Display\nLNI:\nSVIO Select the desired diluted\ninlet (if the option is\ninstalled).\nsent: + SVIO K0 13+\nreceived: + SVIO 0"
          n24 = Increment(x=w89) -> (x+1=w87:i32)
          n25 = Number To Decimal String(number=w87) -> (decimal integer string=w81:string)  [unwired: 1 in]
          n26 = Build Array(w81) -> (w88:string[])
          n27 = call "AK Komm.vi"("Aktionen"=Aktionen_AK_Komm."SVIO", "Daten"=w88) -> ("Empfangsdaten"=w86:string[], "Error"=w84:T37, "Status"=w85:string, "Störung Kommunikation"=w83:bool)  [unwired: 3 in, 3 out]
          n28 = call "Map GD Errors.vi"("Error"=w84, "Störung Kommunikation"=w83) -> ("LIN Errors-Cluster (Ausgang)"=w82:T26)  [unwired: 8 in, 1 out]
        }
        frame 1 {
          # "Analog Display"
          n29 = disable-structure shown="Deaktiviert" {
            frame Disabled {
              n30 = call "AK Komm_ALT.vi"("Aktionen_ALT"=Aktionen_AK_Komm_ALT."EGAK") -> ()  [unwired: 6 in, 5 out]
            }
            frame Enabled {
            }
          }
        }
        frame 2 {
          # "AVL GDU"
          n31 = disable-structure shown="Deaktiviert" {
            frame Disabled {
              n32 = call "AK Komm.vi"("Aktionen"=Aktionen_AK_Komm."EGAK") -> ()  [unwired: 4 in, 7 out]
            }
            frame Enabled {
            }
          }
        }
        frame 3 {
          # "Horiba GDC"
          n33 = disable-structure shown="Deaktiviert" {
            frame Disabled {
              n34 = call "GDC Kom.vi"("Befehl"=Aktion_Befehl."Standby") -> ()  [unwired: 4 in, 7 out]
            }
            frame Enabled {
            }
          }
        }
        frame 4, Default {
          # "HovaCAL, Horiba 710 c"
          n35 = call "FGV_HovaCAL_Interface_GetData.vi"("Aktion"=Aktion_FGV_HovaCAL_Interface_GetData."lesen") -> ("System Cluster out"=w97:T38)  [unwired: 6 in, 4 out]
          n36 = Unbundle By Name(w97) -> ("number of mfc"=w96:i32)
          n37 = Less?(x=w98, y=w96) -> (x < y?=w95:bool)
          n38 = case shown="True" w95 {
            tunnel: w98 -> [_ w101]
            tunnel: [T26 {"Störung Kommunikation"=FALSE, "Pressure carrier gas"=FALSE, "Pressure diluted gas"=FALSE, "Outlet Pressure"=FALSE, "SNOX before SAIR"=FALSE, "Störung Gasteiler"=TRUE} ("LIN Errors-Cluster (Ausgang)") _] -> w94
            frame False {
            }
            frame True {
              n39 = call "FGV_HovaCAL_Interface_AutoLin_MFC.vi"("Aktion"=Aktion_FGV_HovaCAL_Interface_Autolin."schreiben", "AutoLin MFC"=w101) -> ("error out"=w102:errorcluster)  [unwired: 6 in, 3 out]
              n40 = call "SetHovaCAL_MFC_Concentration.vi"("error in (no error)"=w102) -> ()  [unwired: 10 in, 1 out]
            }
          }
        }
        frame 5 {
          # "Horiba 710 c ... manuell !"
        }
      }
      n41 = Concatenate Strings("GD set SPAN to DIL inlet #" ("Status"), w63) -> (w64:string)
      n42 = call "GD TimeStamp.vi"() -> ("date/time string"=w62:string)  [unwired: 10 in, 1 out]
      n43 = Bundle By Name(cluster=T25 {"Wobei"="", "Status"="", "Errors"={"Störung Kommunikation"=FALSE, "Pressure carrier gas"=FALSE, "Pressure diluted gas"=FALSE, "Outlet Pressure"=FALSE, "SNOX before SAIR"=FALSE, "Störung Gasteiler"=FALSE}, "Empfangsdaten"=[], "Zeitstempel"=""} ("GD Info-Cluster in"), "Zeitstempel"=w62, "Wobei"=w64, "Status"=w76, "Errors"=w75, "Empfangsdaten"=w74) -> (w70:T25)
      n44 = call "Status mit GD Info aktualisieren.vi"("show Status even if no Error"=TRUE, "Sprachliste"=w69, "GD Info-Cluster in"=w70) -> ("Status out"=w67:string)  [unwired: 7 in, 1 out]
      "Status out" <- w67
      n45 = call "FGV GD Errors sammeln.vi"("Aktion"=Aktion_FGV_GD_Errors_sammeln."GD Infos sammeln", "GD Info-Cluster in"=w70) -> ()  [unwired: 7 in, 3 out]
      n46 = property class="Str"(reference=w66, "Value"=w67) -> (error out=w68:errorcluster)  [unwired: 1 in, 1 out]
      n47 = call <vilib>:"Clear Errors.vi"("error in (no error)"=w68) -> ()  [unwired: 5 in, 2 out]
    }
  }
  n48 = Unbundle By Name(w14) -> ("Zeitdauer Stufe"=w15:T10, "zusätzliche Zeitdauer Erster Punkt"=w16:sgl)
  n49 = Add(x=w15, y=w16) -> (x+y=w12:T10)
  n50 = Multiply(x=w12, y=T10 1000.0) -> (x*y=w11:T10)
  n51 = disable-structure shown="TestRun==FALSE, Standard" {
    disable-tunnel: w1 -> [_ w105]
    disable-tunnel: [0 ("Analysator Index") w105] -> w5
    frame condition #0 {
      # "#TestRun"
    }
    frame condition #1 (active) {
    }
  }
  n52 = Multiply(x=T10 10.0 ("x*y"), y=T10 1000.0) -> (x*y=w7:T10)
  n53 = case shown="1" w5 {
    tunnel: w25 -> [_ _ _]
    tunnel: w3 -> [_ w142 w216]
    tunnel: w11 -> [_ w141 w215]
    tunnel: w7 -> [_ w140 w214]
    tunnel: "Sprachliste" -> [_ w117 w191]
    tunnel: "Status Str Referenz" -> [_ w112 w186]
    frame 0, Default {
      # "FT-IR"
    }
    frame 1 {
      w121 = T43 {"Wobei"="", "Calibration succesful"=FALSE, "Value is in the valid range"=FALSE, "Zeitstempel"=""} ("Kalibrier Info-Cluster in")
      w108 = "FID E Point" ("Herkunft")
      w109 = "FID 0 Point" ("Herkunft")
      # "FID #GD_Error_TimeStamp"
      n54 = flat-sequence {
        tunnel: w109 -> [w162]
        tunnel: w141 -> [w165]
        tunnel: [w167] -> w137
        tunnel: [w166] -> w134
        tunnel: w109 -> [w172]
        tunnel: [w171] -> w138
        tunnel: w137 -> [w171]
        tunnel: [w170] -> w135
        tunnel: w134 -> [w170]
        tunnel: [w176] -> w139
        tunnel: w138 -> [w176]
        tunnel: [w175] -> w136
        tunnel: w135 -> [w175]
        tunnel: w140 -> [w179]
        tunnel: [w178] -> w126
        tunnel: w139 -> [w178]
        tunnel: [w177] -> w125
        tunnel: w136 -> [w177]
        frame #0 {
          # "GD 0"
          n55 = call "Gasteiler_Nullpunkt.vi"() -> ()  [unwired: 12 in]
        }
        frame #1 {
          # "Zustand"
          n56 = call "FGV-Funktionstasten.vi"("Herkunft"=w162, "Zustand"=Zustaende."Cal-Gas", "Aktion"=Funktionstasten-Aktion."Zustand setzen") -> ()  [unwired: 5 in, 8 out]
        }
        frame #2 {
          # "!!!"
          n57 = Wait Until Next ms Multiple(millisecond multiple=w165) -> ()  [unwired: 1 out]
        }
        frame #3 {
          # "0 Kalibrieren"
          n58 = call "FID Manuell Kalibrieren.vi"("AUTO STARTEN"=TRUE, "Kalibrieren"=FID_Kalibrieren."THC Nullpunkt") -> ("Wert ist im gültigen Bereich:"=w166:bool, "Kalibrieren erfolgreich"=w167:bool)  [unwired: 8 in]
        }
        frame #4 {
          # "Standby ?"
          n59 = call "FGV-Funktionstasten.vi"("Herkunft"=w172, "Zustand"=Zustaende."Standby", "Aktion"=Funktionstasten-Aktion."Zustand setzen") -> ()  [unwired: 5 in, 8 out]
        }
        frame #5 {
          # "GD Standby ?"
          n60 = call "Gasteiler_Standby.vi"() -> ()  [unwired: 12 in]
        }
        frame #6 {
          # "???"
          n61 = Wait Until Next ms Multiple(millisecond multiple=w179) -> ()  [unwired: 1 out]
        }
      }
      n62 = flat-sequence {
        tunnel: w142 -> [w143]
        tunnel: w120 -> [_]
        tunnel: w108 -> [w144]
        tunnel: w141 -> [w147]
        tunnel: [w149] -> w131
        tunnel: [w148] -> w128
        tunnel: w108 -> [w154]
        tunnel: [w153] -> w132
        tunnel: w131 -> [w153]
        tunnel: [w152] -> w129
        tunnel: w128 -> [w152]
        tunnel: [w158] -> w133
        tunnel: w132 -> [w158]
        tunnel: [w157] -> w130
        tunnel: w129 -> [w157]
        tunnel: w140 -> [w161]
        tunnel: [w160] -> w123
        tunnel: w133 -> [w160]
        tunnel: [w159] -> w122
        tunnel: w130 -> [w159]
        frame #0 {
          # "GD0"
          n63 = call "SPAN_Gasteiler_Endpunkt.vi"("Komponente"=w143) -> ()  [unwired: 11 in]
        }
        frame #1 {
          # "Zustand"
          n64 = call "FGV-Funktionstasten.vi"("Herkunft"=w144, "Zustand"=Zustaende."Cal-Gas", "Aktion"=Funktionstasten-Aktion."Zustand setzen") -> ()  [unwired: 5 in, 8 out]
        }
        frame #2 {
          # "!!!"
          n65 = Wait Until Next ms Multiple(millisecond multiple=w147) -> ()  [unwired: 1 out]
        }
        frame #3 {
          w151 = TRUE ("über GT")
          # "E Kalibrieren"
          n66 = call "FID Manuell Kalibrieren.vi"("über GT"=w151, "AUTO STARTEN"=w151, "Kalibrieren"=FID_Kalibrieren."THC Endpunkt") -> ("Wert ist im gültigen Bereich:"=w148:bool, "Kalibrieren erfolgreich"=w149:bool)  [unwired: 7 in]
        }
        frame #4 {
          # "Standby ?"
          n67 = call "FGV-Funktionstasten.vi"("Herkunft"=w154, "Zustand"=Zustaende."Standby", "Aktion"=Funktionstasten-Aktion."Zustand setzen") -> ()  [unwired: 5 in, 8 out]
        }
        frame #5 {
          # "GD Standby ?"
          n68 = call "Gasteiler_Standby.vi"() -> ()  [unwired: 12 in]
        }
        frame #6 {
          # "???"
          n69 = Wait Until Next ms Multiple(millisecond multiple=w161) -> ()  [unwired: 1 out]
        }
      }
      n70 = call "GD TimeStamp.vi"() -> ("date/time string"=w110:string)  [unwired: 10 in, 1 out]
      n71 = Bundle By Name(cluster=w121, "Wobei"=w109, "Calibration succesful"=w126, "Value is in the valid range"=w125, "Zeitstempel"=w110) -> (w119:T43)
      n72 = Bundle By Name(cluster=w121, "Wobei"=w108, "Calibration succesful"=w123, "Value is in the valid range"=w122, "Zeitstempel"=w110) -> (w118:T43)
      n73 = call "FGV GD Errors sammeln.vi"("Aktion"=Aktion_FGV_GD_Errors_sammeln."Kalibrierinfos sammeln", "Kalibrier Info-Cluster in"=w119) -> ("error out"=w120:errorcluster)  [unwired: 7 in, 2 out]
      n74 = call "FGV GD Errors sammeln.vi"("Aktion"=Aktion_FGV_GD_Errors_sammeln."Kalibrierinfos sammeln", "Kalibrier Info-Cluster in"=w118) -> ()  [unwired: 7 in, 3 out]
      n75 = call "Status mit Kalibier Info aktualisieren.vi"("show Status even if no Error"=TRUE, "Sprachliste"=w117, "Kalibrier Info-Cluster in"=w119) -> ("Status out"=w114:string)  [unwired: 7 in, 1 out]
      n76 = call "Status mit Kalibier Info aktualisieren.vi"("show Status even if no Error"=TRUE, "Sprachliste"=w117, "Kalibrier Info-Cluster in"=w118) -> ("Status out"=w113:string)  [unwired: 7 in, 1 out]
      n77 = property class="Str"(reference=w112, "Value"=w114) -> (reference out=w111:refnum<vi>, error out=w116:errorcluster)  [unwired: 1 in]
      n78 = property class="Str"(reference=w111, "Value"=w113) -> (error out=w115:errorcluster)  [unwired: 1 in, 1 out]
      n79 = local write "Status out"(w114) -> ()
      n80 = local write "Status out"(w113) -> ()
      n81 = call <vilib>:"Clear Errors.vi"("error in (no error)"=w116) -> ()  [unwired: 5 in, 2 out]
      n82 = call <vilib>:"Clear Errors.vi"("error in (no error)"=w115) -> ()  [unwired: 5 in, 2 out]
    }
    frame 2 {
      w198 = T43 {"Wobei"="", "Calibration succesful"=FALSE, "Value is in the valid range"=FALSE, "Zeitstempel"=""} ("Kalibrier Info-Cluster in")
      w182 = "PMA E Point" ("Herkunft")
      w183 = "PMA 0 Point" ("Herkunft")
      # "PMA #GD_Error_TimeStamp"
      n83 = flat-sequence {
        tunnel: w183 -> [w237]
        tunnel: w215 -> [w240]
        tunnel: [w242] -> w211
        tunnel: [w241] -> w208
        tunnel: w183 -> [w247]
        tunnel: [w246] -> w212
        tunnel: w211 -> [w246]
        tunnel: [w245] -> w209
        tunnel: w208 -> [w245]
        tunnel: [w251] -> w213
        tunnel: w212 -> [w251]
        tunnel: [w250] -> w210
        tunnel: w209 -> [w250]
        tunnel: w214 -> [w254]
        tunnel: [w253] -> w199
        tunnel: w213 -> [w253]
        tunnel: [w252] -> w195
        tunnel: w210 -> [w252]
        frame #0 {
          # "GD 0"
          n84 = call "Gasteiler_Nullpunkt.vi"() -> ()  [unwired: 12 in]
        }
        frame #1 {
          # "Zustand"
          n85 = call "FGV-Funktionstasten.vi"("Herkunft"=w237, "Zustand"=Zustaende."Cal-Gas", "Aktion"=Funktionstasten-Aktion."Zustand setzen") -> ()  [unwired: 5 in, 8 out]
        }
        frame #2 {
          # "!!!"
          n86 = Wait Until Next ms Multiple(millisecond multiple=w240) -> ()  [unwired: 1 out]
        }
        frame #3 {
          # "0 Kalibrieren"
          n87 = call "PMA Manuell Kalibrieren.vi"("Kalibrieren"=Kalibrierung_O2."Nullpunkt O2", "AUTO STARTEN"=TRUE) -> ("Wert im gültigen Bereich:"=w241:bool, "Kalibrieren erfolgreich"=w242:bool)  [unwired: 8 in]
        }
        frame #4 {
          # "Standby ?"
          n88 = call "FGV-Funktionstasten.vi"("Herkunft"=w247, "Zustand"=Zustaende."Standby", "Aktion"=Funktionstasten-Aktion."Zustand setzen") -> ()  [unwired: 5 in, 8 out]
        }
        frame #5 {
          # "GD Standby ?"
          n89 = call "Gasteiler_Standby.vi"() -> ()  [unwired: 12 in]
        }
        frame #6 {
          # "???"
          n90 = Wait Until Next ms Multiple(millisecond multiple=w254) -> ()  [unwired: 1 out]
        }
      }
      n91 = flat-sequence {
        tunnel: w216 -> [w217]
        tunnel: w194 -> [_]
        tunnel: w182 -> [w218]
        tunnel: w215 -> [w221]
        tunnel: [w223] -> w205
        tunnel: [w222] -> w202
        tunnel: w182 -> [w229]
        tunnel: [w228] -> w206
        tunnel: w205 -> [w228]
        tunnel: [w227] -> w203
        tunnel: w202 -> [w227]
        tunnel: [w233] -> w207
        tunnel: w206 -> [w233]
        tunnel: [w232] -> w204
        tunnel: w203 -> [w232]
        tunnel: w214 -> [w236]
        tunnel: [w235] -> w197
        tunnel: w207 -> [w235]
        tunnel: [w234] -> w196
        tunnel: w204 -> [w234]
        frame #0 {
          # "GD0"
          n92 = call "SPAN_Gasteiler_Endpunkt.vi"("Komponente"=w217) -> ()  [unwired: 11 in]
        }
        frame #1 {
          # "Zustand"
          n93 = call "FGV-Funktionstasten.vi"("Herkunft"=w218, "Zustand"=Zustaende."Cal-Gas", "Aktion"=Funktionstasten-Aktion."Zustand setzen") -> ()  [unwired: 5 in, 8 out]
        }
        frame #2 {
          # "!!!"
          n94 = Wait Until Next ms Multiple(millisecond multiple=w221) -> ()  [unwired: 1 out]
        }
        frame #3 {
          # "E Kalibrieren"
          n95 = call "PMA Manuell Kalibrieren.vi"("GT"=TRUE, "Kalibrieren"=Kalibrierung_O2."Endpunkt O2", "AUTO STARTEN"=TRUE) -> ("Wert im gültigen Bereich:"=w222:bool, "Kalibrieren erfolgreich"=w223:bool)  [unwired: 7 in]
        }
        frame #4 {
          # "Standby ?"
          n96 = call "FGV-Funktionstasten.vi"("Herkunft"=w229, "Zustand"=Zustaende."Standby", "Aktion"=Funktionstasten-Aktion."Zustand setzen") -> ()  [unwired: 5 in, 8 out]
        }
        frame #5 {
          # "GD Standby ?"
          n97 = call "Gasteiler_Standby.vi"() -> ()  [unwired: 12 in]
        }
        frame #6 {
          # "???"
          n98 = Wait Until Next ms Multiple(millisecond multiple=w236) -> ()  [unwired: 1 out]
        }
      }
      n99 = call "GD TimeStamp.vi"() -> ("date/time string"=w184:string)  [unwired: 10 in, 1 out]
      n100 = Bundle By Name(cluster=w198, "Wobei"=w183, "Calibration succesful"=w199, "Value is in the valid range"=w195, "Zeitstempel"=w184) -> (w193:T43)
      n101 = Bundle By Name(cluster=w198, "Wobei"=w182, "Calibration succesful"=w197, "Value is in the valid range"=w196, "Zeitstempel"=w184) -> (w192:T43)
      n102 = call "FGV GD Errors sammeln.vi"("Aktion"=Aktion_FGV_GD_Errors_sammeln."Kalibrierinfos sammeln", "Kalibrier Info-Cluster in"=w193) -> ("error out"=w194:errorcluster)  [unwired: 7 in, 2 out]
      n103 = call "FGV GD Errors sammeln.vi"("Aktion"=Aktion_FGV_GD_Errors_sammeln."Kalibrierinfos sammeln", "Kalibrier Info-Cluster in"=w192) -> ()  [unwired: 7 in, 3 out]
      n104 = call "Status mit Kalibier Info aktualisieren.vi"("show Status even if no Error"=TRUE, "Sprachliste"=w191, "Kalibrier Info-Cluster in"=w193) -> ("Status out"=w188:string)  [unwired: 7 in, 1 out]
      n105 = call "Status mit Kalibier Info aktualisieren.vi"("show Status even if no Error"=TRUE, "Sprachliste"=w191, "Kalibrier Info-Cluster in"=w192) -> ("Status out"=w187:string)  [unwired: 7 in, 1 out]
      n106 = property class="Str"(reference=w186, "Value"=w188) -> (reference out=w185:refnum<vi>, error out=w190:errorcluster)  [unwired: 1 in]
      n107 = property class="Str"(reference=w185, "Value"=w187) -> (error out=w189:errorcluster)  [unwired: 1 in, 1 out]
      n108 = local write "Status out"(w188) -> ()
      n109 = local write "Status out"(w187) -> ()
      n110 = call <vilib>:"Clear Errors.vi"("error in (no error)"=w190) -> ()  [unwired: 5 in, 2 out]
      n111 = call <vilib>:"Clear Errors.vi"("error in (no error)"=w189) -> ()  [unwired: 5 in, 2 out]
    }
  }
  "error out" <- "error in (no error)"
  "SPAN Index out" <- "SPAN Index"
  "SpanInletClusterArray out" <- "SpanInletClusterArray"
